vi "Command DUT Stop Processes.vi"(8 "error in (no error)":errorcluster, 11 "DUT Sample in":refnum<class "DUT Sample.lvclass">) -> (0 "error out":errorcluster, 3 "DUT Sample out":refnum<class "DUT Sample.lvclass">)   [LabVIEW 2023, in "DUT Sample.lvclass"]
uses:
  DUT Sample.lvclass
  DUT Sample.lvclass/DUT Sample.ctl
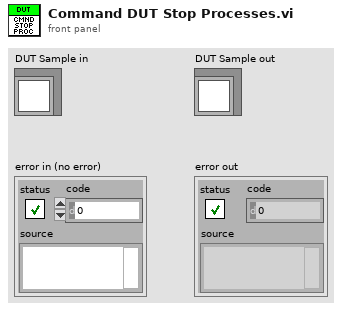
[diagram p1: front panel]
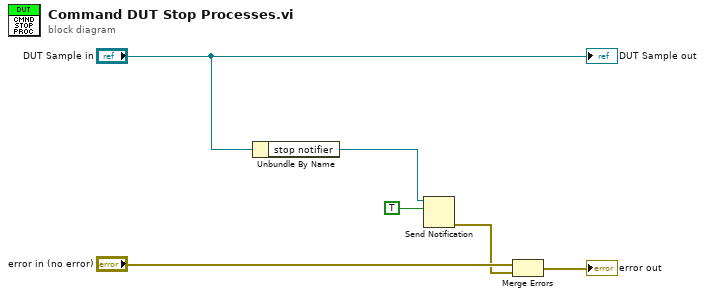
[diagram p0: block diagram]
diagram:
  n1 = Unbundle By Name("DUT Sample in") -> ("stop notifier"=w4:refnum<notifier>)
  n2 = Send Notification(notification=TRUE, notifier=w4) -> (error out=w1:errorcluster)  [unwired: 1 in, 1 out]
  n3 = Merge Errors("error in (no error)", w1) -> (→"error out":errorcluster)
  "DUT Sample out" <- "DUT Sample in"
